vi "Main Chroma 19053 hipot.vi"   [LabVIEW 2018]
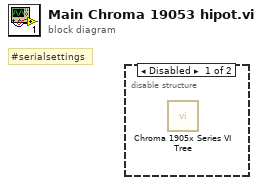
[diagram p0: block diagram]
diagram:
  # "#serialsettings"
  n1 = disable-structure shown="Disabled" {
    frame Disabled {
      n2 = call <instrlib>:"Chroma 1905x Series VI Tree.vi"() -> ()  [unwired: 1 in]
    }
    frame Enabled {
    }
  }
